vi "Read Msg Ref.vi"(7 "Actor":refnum<class "Actor.lvclass">) -> (2 "Msg Ref":refnum<event-registration>)   [LabVIEW 2025, in "jettl.lvlib" / "Transport.lvlib" / "Event.lvlib"]
uses:
  Event.lvlib
  Actor/Actor/Actor.lvclass
  Msg/Msg.lvclass
  Event Transport/Event Transport.lvclass
  Attributes/Attributes/Attributes.lvclass
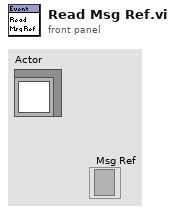
[diagram p1: front panel]
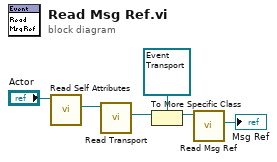
[diagram p0: block diagram]
diagram:
  n1 = call-dynamic "Read Self Attributes.vi"("Actor in"="Actor") -> ("Self Attributes"=w6:refnum<class "Attributes.lvclass">)  [unwired: 10 in]
  n2 = call-dynamic "Read Transport.vi"("Attributes in"=w6) -> ("Transport"=w3:refnum<class "Transport.lvclass">)  [unwired: 10 in]
  n3 = To More Specific Class(target class=refnum<class "Event Transport.lvclass"> refnum ("jettl.lvlib:Transport.lvlib:Event Transport.lvclass"), reference=w3) -> (specific class reference=w2:refnum<class "Event Transport.lvclass">)  [unwired: 1 in, 1 out]
  n4 = call "Read Msg Ref.vi"("Event Transport in"=w2) -> ("Msg Ref"=→"Msg Ref":refnum<event-registration>)  [unwired: 10 in]
